vi "RWA_Read Section from File.vi"(8 "Error":errorcluster, 9 "Section Name":string, 11 "Path":path) -> (0 "Error Out":errorcluster, 1 "Found? Out":bool, 2 "Section String Out":string, 3 "Duplicate Path Out":path)   [LabVIEW 2020]
doc: "This VI was created for use with the Read/Write Anything VIs. It reads all the keys and their values from the specified section.\n\nAuthored by Robert C. Mortensen\nsupport@mooregoodideas.com\nwww.mooregoodideas.com\n\nCopyright (c) 2010, Moore Good Ideas, Inc.\n\nAll rights reserved.\n\nRedistribution and use in source and binary forms, with or without modification, are permitted provided that the following conditions are met:\n\n * Redistributions of source code must retain the above copyright notice, this list of conditions and the following disclaimer.\n * Redistributions in binary form must reproduce the above copyright notice, this list of conditions and the following disclaimer in the documentation and/or other materials provided with the distribution.\n * Neither the name of Moore Good Ideas, Inc. nor the names of its contributors may be used to endorse or promote products derived from this software without specific prior written permission.\n\nTHIS SOFTWARE IS PROVIDED BY THE COPYRIGHT HOLDERS AND CONTRIBUTORS \"AS IS\" AND ANY EXPRESS OR IMPLIED WARRANTIES, INCLUDING, BUT NOT LIMITED TO, THE IMPLIED WARRANTIES OF MERCHANTABILITY AND FITNESS FOR A PARTICULAR PURPOSE ARE DISCLAIMED. IN NO EVENT SHALL THE COPYRIGHT OWNER OR CONTRIBUTORS BE LIABLE FOR ANY DIRECT, INDIRECT, INCIDENTAL, SPECIAL, EXEMPLARY, OR CONSEQUENTIAL DAMAGES (INCLUDING, BUT NOT LIMITED TO, PROCUREMENT OF SUBSTITUTE GOODS OR SERVICES; LOSS OF USE, DATA, OR PROFITS; OR BUSINESS INTERRUPTION) HOWEVER CAUSED AND ON ANY THEORY OF LIABILITY, WHETHER IN CONTRACT, STRICT LIABILITY, OR TORT (INCLUDING NEGLIGENCE OR OTHERWISE) ARISING IN ANY WAY OUT OF THE USE OF THIS SOFTWARE, EVEN IF ADVISED OF THE POSSIBILITY OF SUCH DAMAGE."
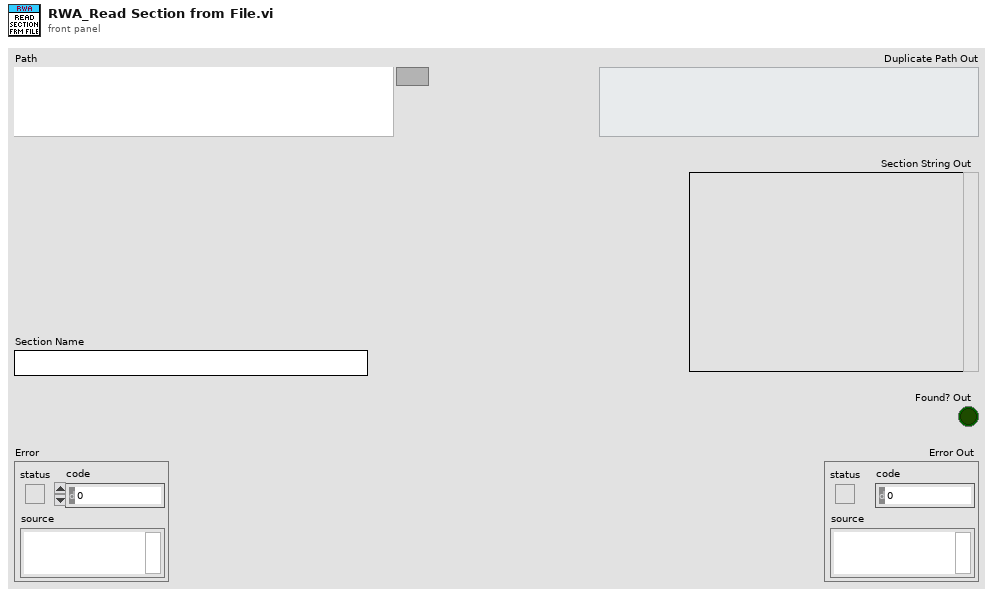
[diagram p1: front panel]
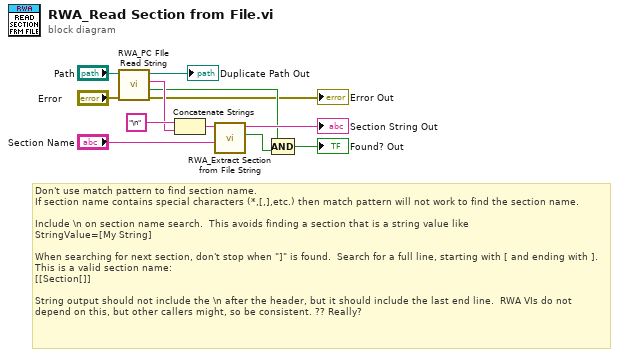
[diagram p0: block diagram]
diagram:
  # "Don't use match pattern to find section name.\nIf section name contains special characters (*,[,],etc.) then match pattern will not work to find the section name.\n\nInclude \\n on section name search.  This avoids finding a section that is a string value like\nStringValue=[My String]\n\nWhen searching for next section, don't stop when \"]\" is found.  Search for a full line, starting with [ and ending with ].  This is a valid section name:\n[[Section[]]\n\nString output should not include the \\n after the header, but it should include the last end line.  RWA VIs do not depend on this, but other callers might, so be consistent. ?? Really?"
  n1 = call "RWA_PC FIle Read String.vi"("Error"="Error", "Path"="Path") -> ("Error Out"=→"Error Out":errorcluster, "Found"=w2:bool, "String Out"=w6:string, "Duplicate Path Out"=→"Duplicate Path Out":path)  [unwired: 6 in]
  n2 = Concatenate Strings("\n" ("string"), w6) -> (w11:string)
  n3 = call "RWA_Extract Section from File String.vi"("Section Name"="Section Name", "String"=w11) -> ("Found? Out"=w8:bool, "String Out"=→"Section String Out":string)  [unwired: 8 in]
  n4 = Compound Arithmetic op=AND(w2, w8) -> (→"Found? Out":bool)
